vi "Prepare XY graph.vi"(9 "col2":i32, 10 "col1":i32, 11 "Array":dbl[][](array[numeric])) -> (3 "XY":cluster{dbl[], dbl[]})   [LabVIEW 2023]
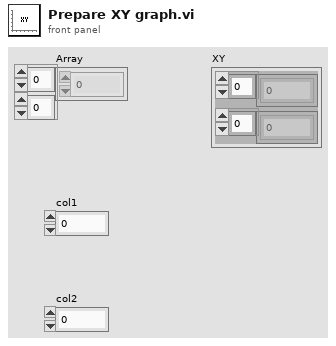
[diagram p1: front panel]
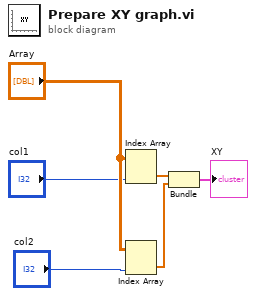
[diagram p0: block diagram]
diagram:
  n1 = Index Array(array="Array", index (col)="col1") -> (element=w5:dbl[])  [unwired: 1 in]
  n2 = Index Array(array="Array", index (col)="col2") -> (element=w2:dbl[])  [unwired: 1 in]
  n3 = Bundle("Array"=w5, "Array"=w2) -> (→"XY":cluster{"Array":dbl[], "Array":dbl[]})  [unwired: 1 in]
